vi "GCS26.vi"() -> ()   [LabVIEW 2009]
uses:
  <vilib>/robotics/Controls/Attitude Indicator/Attitude Indicator.xctl
  <vilib>/robotics/Controls/Compass Indicator/Compass Indicator.xctl
  <vilib>/Instr/_visa.llb/VISA Set IO Buffer Mask.ctl
  <vilib>/Instr/_visa.llb/VISA Configure Serial Port (Instr).vi
  user32.dll
panel:
  out "Current Time":string
  out "Compass Indicator":dbl(xcontrol)
  out "Attitude Indicator":cluster{"Roll":dbl, "Pitch":dbl}(xcontrol)
  out "Autopilot switch":bool
  in  "EARTHLib.IKHInterface":refnum<k7>
  out "OriginalChild":i32
  out "TRUE SPEED":dbl(knob) scale=0.0..120.0
  out "COURSE/BEARING":cluster{i16, i16}(knob) scale=0.0..360.0 scale format="%.0f°"
  out "Distance To WP":i32
  out "Current WP":i32
  out "Altitude":cluster{i32, i32}(knob) scale=0.0..200.0
  in  "WebBrowser":refnum<k7>(container)
  out "Air Speed":i32 format="%.0f m/s"
  out "Pitch":i32
  out "Roll":i32
  out "Lat":dbl format="%.6g°"
  out "Lon":dbl format="%.6g°"
  out "Ground Speed":i32 format="%.0f m/s"
  out "C/S Rate\n     Rate":sgl(knob) scale=-5.0..5.0 scale format="%#.2g"
  out "AirSpeed":cluster{i16, i16}(knob)={0, 31} scale=0.0..40.0
  out "Amps":dbl format="%.2f"
  out "Est Time Left":dbl(knob) min=0.0 max=0.0 scale=0.0..60.0 scale format="%#_2f"
  in  "Launch EXE":bool
  out "Watts":dbl format="%.2f"
  out "Slide":u8(slide) scale=0.0..100.0
  out "Throttle S.P":i32 format="%.0f of 100%"
  out "Battery Voltage":dbl format="%#_g V"
  out "LIPO":sgl(slide) scale=9.0..12.6 scale format="%#_g V"
  in  "Logging":bool
  in  "quit?":bool
  in  "Amps FT":i32=34
  in  "MAh's":dbl=2100.0
  in  "Cell Count":dbl=3.0 format="%#_4g"
  out "Boolean 2":bool
  out "Boolean":bool
  in  "Speed":bool
  in  "Baud Rate":string(combo)="38400"
  in  "Choose Port":refnum<visa-resource-name>
  out "error out":errorcluster
  out "Part2":string
  out "Part1":string
  out "ALT":string
  out "originalParent":u32
  in  "EARTHLib.IApplicationGE":refnum<k7>
  in  "WaitForExit":bool
  out "Numeric":i32
  # "C/S Rate"
  # "Air Speed"
  # "Time Left"
  # "Throttle S.P"
  # "LIPO CONDITION"
  # "DIYdrones.com\nEasyuav.com"
  # "ALTITUDE"
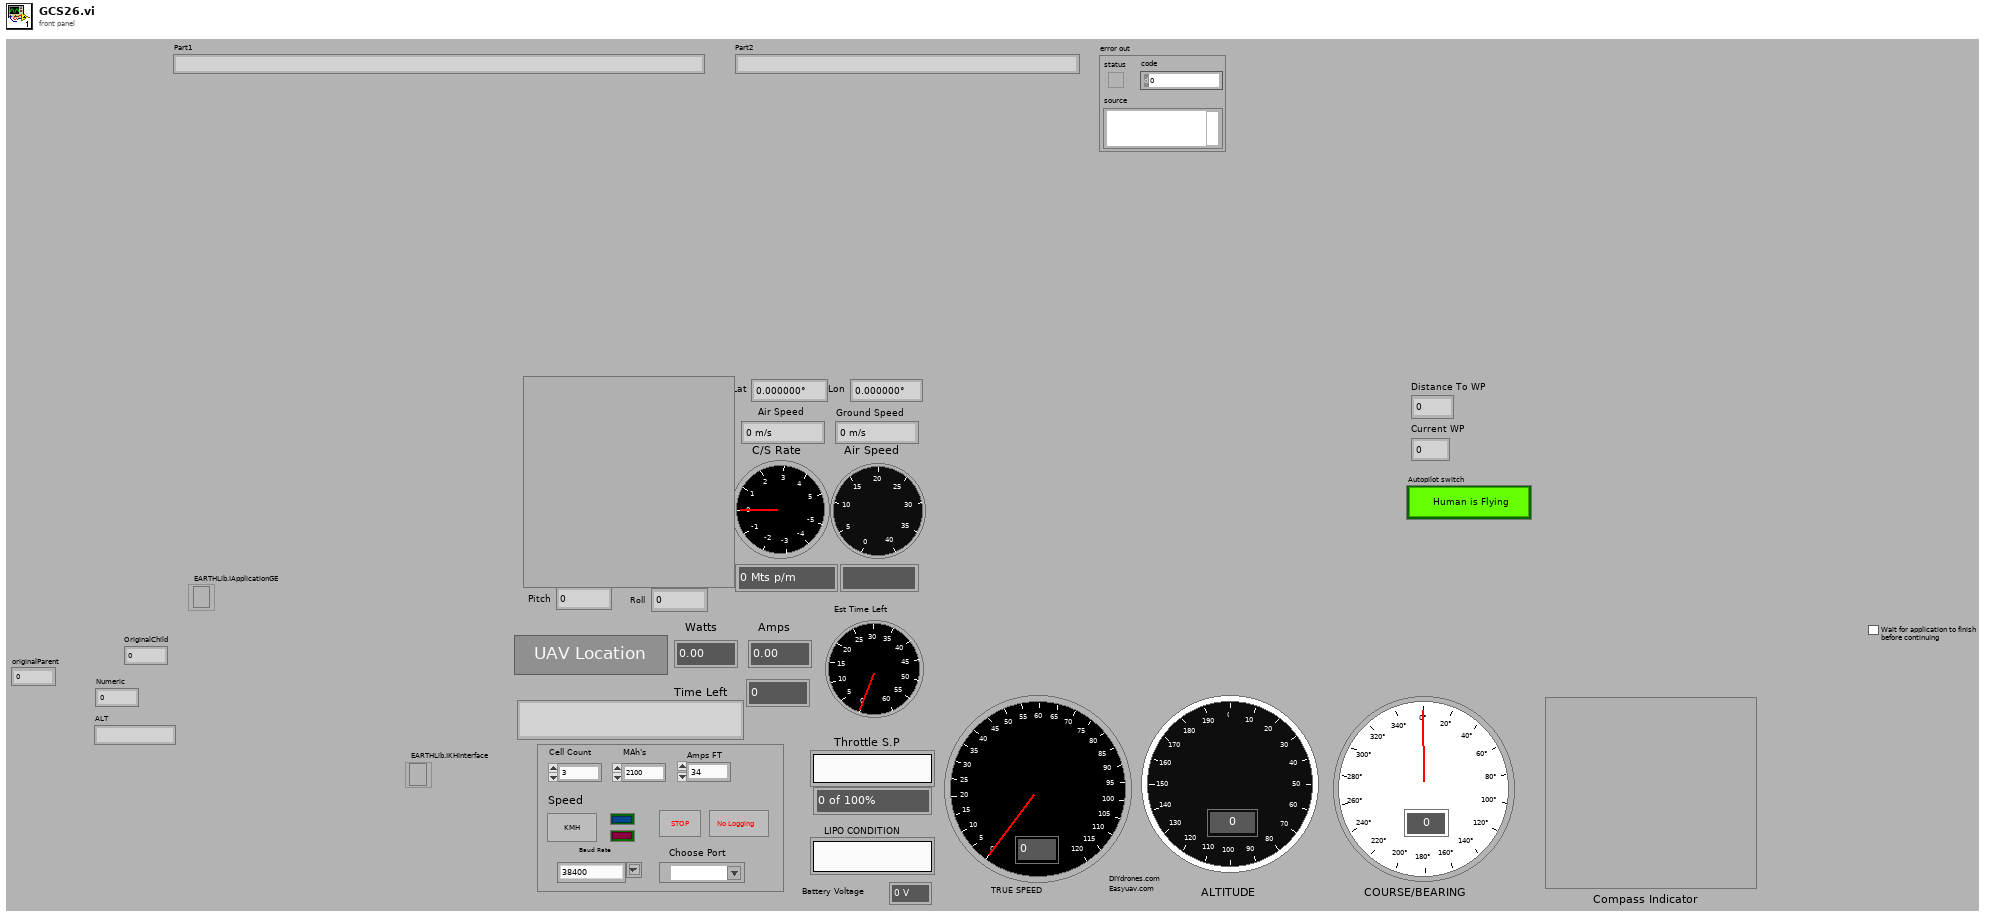
[diagram p1: front panel]
types:
  T1 = enum16{"open", "replace", "create", "open or create", "replace or create", "replace or create with confirmation"}
  T2 = typedef "VISA Set IO Buffer Mask.ctl" = u16
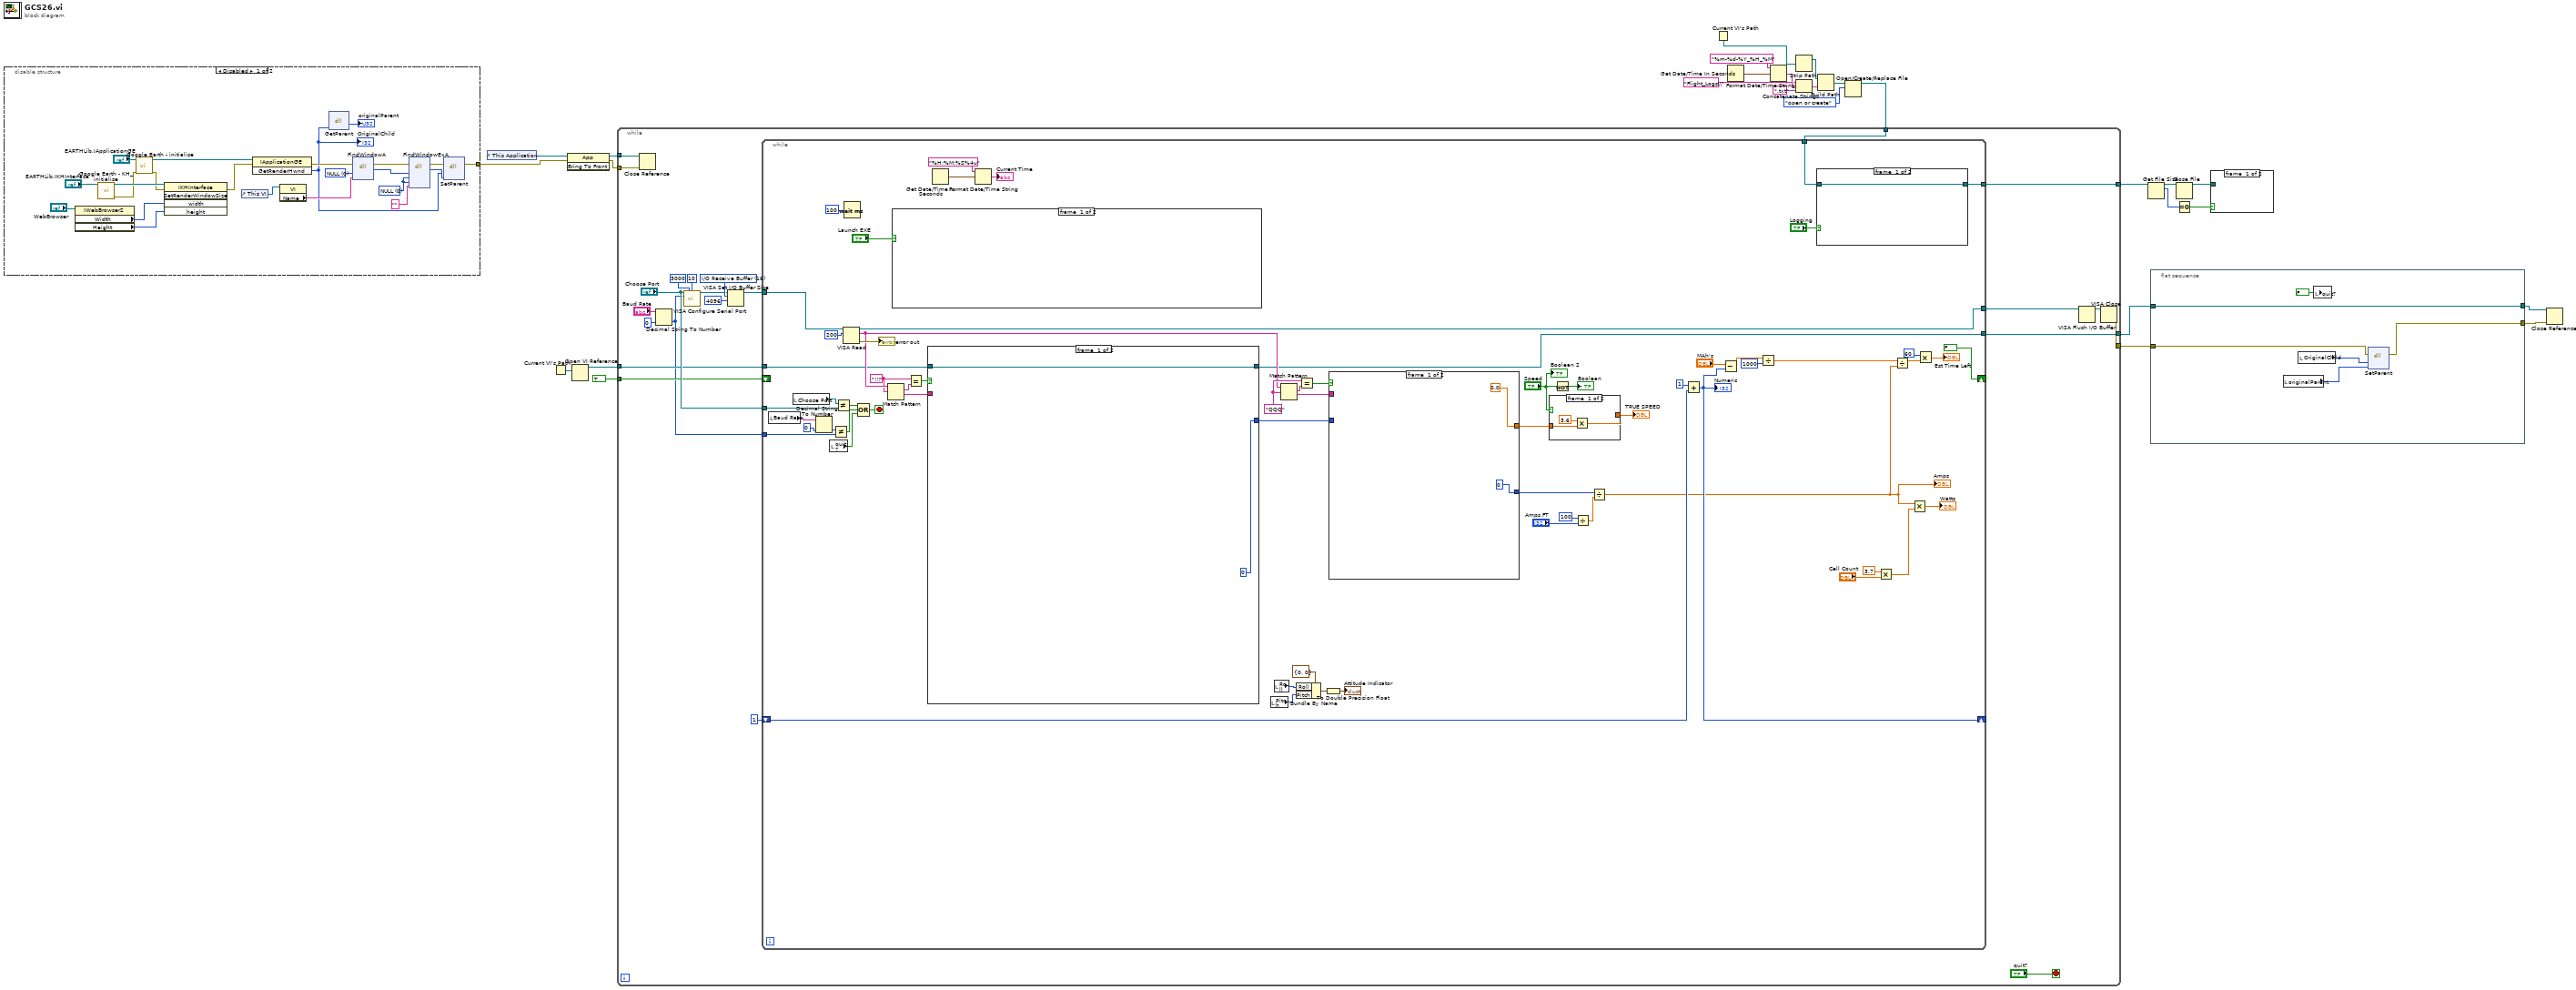
[diagram p0: block diagram]
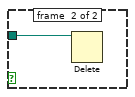
[diagram p2: hidden frame]
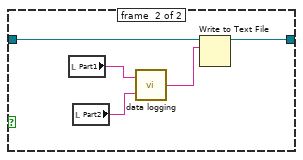
[diagram p4: hidden frame]
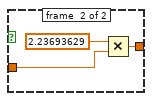
[diagram p5: hidden frame]
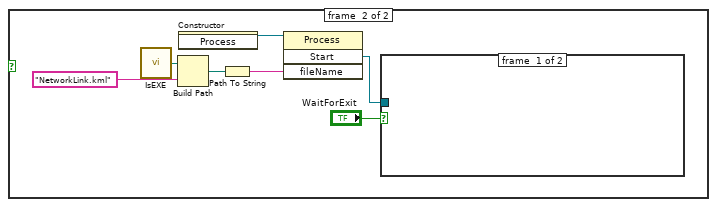
[diagram p6: hidden frame]
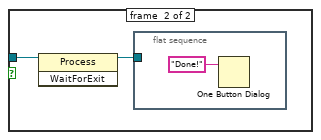
[diagram p7: hidden frame]
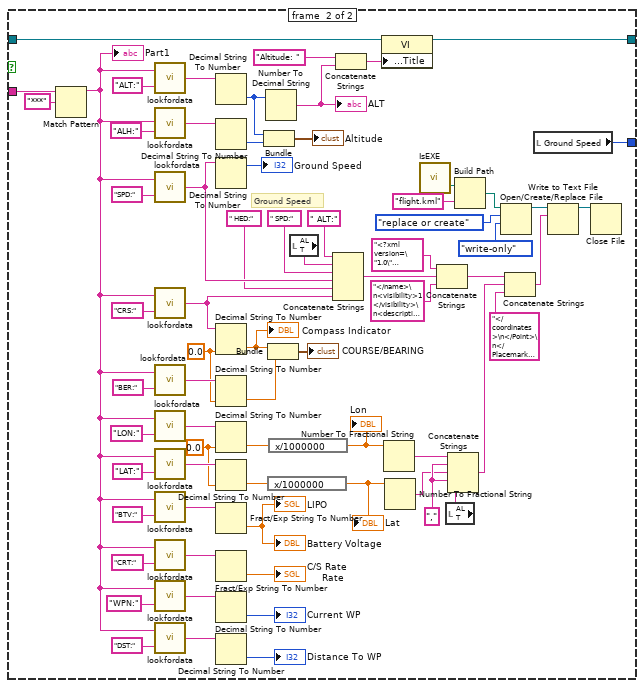
[diagram p8: hidden frame]
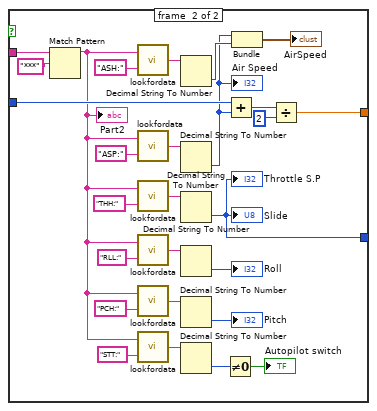
[diagram p9: hidden frame]
diagram:
  n1 = disable-structure shown="Disabled" {
    disable-tunnel: [w29 _] -> w7
    frame #0 {
      w46 = 0 items=["NULL"]
      w48 = 0 items=["NULL"]
      n2 = property class="IWebBrowser2"(reference="WebBrowser") -> ("Width"=w33:i32, "Height"=w32:i32)  [unwired: 1 in, 2 out]
      n3 = call "Google Earth - KH_initialise.vi"("EARTHLib.IKHInterface"="EARTHLib.IKHInterface") -> ("error out"=w28:errorcluster, "Refnum Out"=w34:refnum<k7>)  [unwired: 1 in, 8 out]
      n4 = call "Google Earth - initialise.vi"("error in (no error)"=w28, "EARTHLib.IApplicationGE"="EARTHLib.IApplicationGE") -> ("error out"=w31:errorcluster, "Refnum Out"=w49:refnum<k7>)  [unwired: 8 out]
      n5 = invoke class="IKHInterface" method="SetRenderWindowSize"(reference=w34, error in=w31, "width"=w33, "height"=w32) -> (error out=w30:errorcluster)  [unwired: 1 in, 4 out]
      n6 = control-ref of="This VI"() -> (w40:refnum<vi>)
      n7 = invoke class="IApplicationGE" method="GetRenderHwnd"(reference=w49, error in=w30) -> (error out=w37:errorcluster, "GetRenderHwnd"=w36:i32)  [unwired: 1 in, 1 out]
      "OriginalChild" <- w36
      n8 = property class="VI"(reference=w40) -> ("Name"=w39:string)  [unwired: 1 in, 2 out]
      n9 = dll-call lib="user32.dll" fn="GetParent" label="Get Parent"("hWndChild"=w36) -> ("hWnd"=→"originalParent":u32)  [unwired: 4 in, 2 out]
      n10 = dll-call lib="user32.dll" fn="FindWindowA" label="FindWindow"(error in=w37, "lpszClassName"=w48, "lpszWindowName"=w39) -> (error out=w43:errorcluster, "hWnd"=w47:u32)  [unwired: 4 in, 1 out]
      n11 = dll-call lib="user32.dll" fn="FindWindowExA" label="Find Child"(error in=w43, "Parent HWND"=w47, "Child_After HWND"=w46, "lpszClassName"=w46, "lpszWindowName"="") -> (error out=w41:errorcluster, "hWnd"=w45:u32)  [unwired: 5 in, 2 out]
      n12 = dll-call lib="user32.dll" fn="SetParent" label="Set Parent"(error in=w41, "hWndChild"=w36, "hWndNewParent"=w45) -> (error out=w29:errorcluster)  [unwired: 4 in, 2 out]
    }
    frame #1 {
    }
  }
  n13 = control-ref of="This Application"() -> (w20:refnum<vi>)
  n14 = Current VI's Path() -> (path=w26:path)
  n15 = invoke class="App" method="Bring To Front"(reference=w20, error in=w7) -> (reference out=w19:refnum<vi>, error out=w18:errorcluster)  [unwired: 1 in, 1 out]
  n16 = Open VI Reference(vi path=w26) -> (vi reference=w25:refnum<vi>)  [unwired: 1 in, 5 out]
  n17 = Current VI's Path() -> (path=w9:path)
  n18 = Get Date/Time In Seconds() -> (seconds since 1Jan1904=w12:timestamp)
  n19 = Format Date/Time String(time format string (%c)="%m-%d-%Y_%H_%M", seconds (now)=w12) -> (date/time string=w11:string)  [unwired: 1 out]
  n20 = Strip Path(path=w9) -> (stripped path=w8:path)  [unwired: 1 out]
  n21 = Concatenate Strings("Flight_Logs\\" ("string"), w11, ".txt" ("string")) -> (w17:string)
  n22 = Build Path(base path=w8, name or relative path=w17) -> (appended path=w15:path)
  n23 = Open/Create/Replace File(file path (use dialog)=w15, operation (0:open)=T1."open or create") -> (refnum out=w14:refnum<file>)  [unwired: 1 in, 5 out]
  n24 = while {
    tunnel: TRUE -> [w63]
    tunnel: [w62] -> w24
    tunnel: w25 -> [w61]
    tunnel: [w57] -> w21
    tunnel: w19 -> [w56]
    tunnel: w18 -> [w55]
    tunnel: [w54] -> w5
    tunnel: w14 -> [w53]
    stop <- "quit?" stop-if-true
    w72 = T2 16 items=["I/O Receive Buffer"=16, "I/O Transmit Buffer"=32, "I/O Receive and Transmit Buffer"=48] ("Mask")
    n25 = Close Reference(reference=w56, error in (no error)=w55) -> ()  [unwired: 1 out]
    n26 = Decimal String To Number(string="Baud Rate", default (0L)=u32 0 ("default (0 I32)")) -> (number=w52:u32)  [unwired: 2 out]
    n27 = call-poly "VISA Configure Serial Port"("VISA resource name"="Choose Port", "timeout (10sec)"=u32 3000, "termination char\n(0xA = '\\n' = LF)"=u8 10 ("termination char\n(0xA = '\\n' = LF)"), "baud rate (9600)"=w52) -> ("VISA resource name out"=w65:refnum<visa-resource-name>)  [unwired: 5 in, 6 out]
    n28 = VISA Set I/O Buffer Size(VISA resource name=w65, mask (16)=w72, size (4096)=u32 4096) -> (VISA resource name out=w70:refnum<visa-resource-name>)  [unwired: 1 in, 1 out]
    n29 = while {
      tunnel: w70 -> [w134]
      tunnel: [w133] -> w69
      tunnel: "Choose Port" -> [w123]
      shift-right: [FALSE] -> _
      shift-left: w63 -> [_]
      tunnel: [w121] -> w62
      tunnel: w61 -> [w120]
      tunnel: w52 -> [w119]
      shift-right: [w102] -> _
      shift-left: 1 ("Slide 2") -> [w113]
      tunnel: [w88] -> w54
      tunnel: w53 -> [w87]
      stop <- w116 stop-if-true
      w128 = "QQQ" ("regular expression")
      w76 = "!!!" ("regular expression")
      n30 = local read "Baud Rate"() -> (w115:string)
      n31 = local read "Choose Port"() -> (w124:refnum<visa-resource-name>)
      n32 = Decimal String To Number(string=w115, default (0L)=u32 0 ("default (0 I32)")) -> (number=w74:u32)  [unwired: 2 out]
      n33 = local read "quit?"() -> (w90:bool)
      n34 = Not Equal?(x=w74, y=w119) -> (x != y?=w117:bool)
      n35 = Not Equal?(x=w124, y=w123) -> (x != y?=w118:bool)
      n36 = VISA Read(VISA resource name=w134, byte count=u32 200) -> (VISA resource name out=w133:refnum<visa-resource-name>, read buffer=w126:string, error out=→"error out":errorcluster)  [unwired: 1 in, 1 out]
      n37 = Wait (ms)(milliseconds to wait=u32 100) -> ()  [unwired: 1 out]
      n38 = Compound Arithmetic op=OR(w118, w117, w90) -> (w116:bool)
      n39 = Match Pattern(string=w126, regular expression=w76) -> (match substring=w75:string, after substring=w135:string)  [unwired: 3 out]
      n40 = case shown="True" "Launch EXE" {
        frame #0 {
        }
        frame #1 {
          n41 = call "IsEXE.vi"() -> ("path to vi or exe install\\data\\ dir"=w148:path)  [unwired: 10 out]
          n42 = Build Path(base path=w148, name or relative path="NetworkLink.kml") -> (appended path=w149:path)
          n43 = constructor class="Process"() -> (reference out=w154:refnum<k24>)  [unwired: 3 in, 2 out]
          n44 = Path To String(path=w149) -> (string=w153:string)
          n45 = invoke class="Process" method="Start"(reference=w154, "fileName"=w153) -> ("Start"=w152:refnum<k24>)  [unwired: 2 in, 3 out]
          n46 = case shown="True" "WaitForExit" {
            tunnel: w152 -> [_ w156]
            frame #0 {
            }
            frame #1 {
              n47 = invoke class="Process" method="WaitForExit"(reference=w156) -> (reference out=w155:refnum<k24>)  [unwired: 2 in, 2 out]
              n48 = flat-sequence {
                tunnel: w155 -> [_]
                frame #0 {
                  n49 = One Button Dialog(message="Done!") -> ()  [unwired: 2 out]
                }
              }
            }
          }
        }
      }
      n50 = Equal?(x=w76, y=w75) -> (x = y?=w106:bool)
      n51 = case shown="True" w106 {
        tunnel: w135 -> [_ w187]
        tunnel: [w158 w184] -> w121
        tunnel: w120 -> [w158 w161]
        tunnel: [0 ("Numeric") w173] -> w112
        frame #0 {
        }
        frame #1 {
          w162 = 0.0 ("default (0 I32)")
          w163 = 0.0 ("default (0 I32)")
          w176 = ","
          # "Ground Speed"
          n52 = Match Pattern(string=w187, regular expression="***") -> (before substring=w168:string)  [unwired: 4 out]
          "Part1" <- w168
          n53 = call "lookfordata.vi"("Header"="ALT:" ("regular expression"), "string"=w168) -> ("output string"=w160:string)
          n54 = call "lookfordata.vi"("Header"="ALH:" ("regular expression"), "string"=w168) -> ("output string"=w225:string)
          n55 = call "lookfordata.vi"("Header"="SPD:", "string"=w168) -> ("output string"=w194:string)
          n56 = call "lookfordata.vi"("Header"="CRS:", "string"=w168) -> ("output string"=w191:string)
          n57 = call "lookfordata.vi"("Header"="BER:", "string"=w168) -> ("output string"=w223:string)
          n58 = call "lookfordata.vi"("Header"="LON:", "string"=w168) -> ("output string"=w213:string)
          n59 = call "lookfordata.vi"("Header"="LAT:", "string"=w168) -> ("output string"=w211:string)
          n60 = call "lookfordata.vi"("Header"="BTV:", "string"=w168) -> ("output string"=w181:string)
          n61 = call "lookfordata.vi"("Header"="CRT:", "string"=w168) -> ("output string"=w189:string)
          n62 = call "lookfordata.vi"("Header"="WPN:", "string"=w168) -> ("output string"=w219:string)
          n63 = call "lookfordata.vi"("Header"="DST:", "string"=w168) -> ("output string"=w209:string)
          n64 = Decimal String To Number(string=w160) -> (number=w178:i32)  [unwired: 3 out]
          n65 = Decimal String To Number(string=w225) -> (number=w226:i32)  [unwired: 3 out]
          n66 = Decimal String To Number(string=w194) -> (offset past number=→"Ground Speed":i32)  [unwired: 3 out]
          n67 = Decimal String To Number(string=w191, default (0L)=w162) -> (number=w166:dbl)  [unwired: 2 out]
          "Compass Indicator" <- w166
          n68 = Decimal String To Number(string=w223, default (0L)=w162) -> (number=w224:dbl)  [unwired: 2 out]
          n69 = Decimal String To Number(string=w213, default (0L)=w163) -> (number=w165:dbl)  [unwired: 2 out]
          n70 = Decimal String To Number(string=w211, default (0L)=w163) -> (number=w164:dbl)  [unwired: 2 out]
          n71 = Fract/Exp String To Number(string=w181) -> (number=→"LIPO" →"Battery Voltage":dbl)  [unwired: 4 out]
          n72 = Fract/Exp String To Number(string=w189) -> (number=→"C/S Rate\n     Rate":dbl)  [unwired: 4 out]
          n73 = Decimal String To Number(string=w219) -> (number=→"Current WP":i32)  [unwired: 3 out]
          n74 = Decimal String To Number(string=w209) -> (number=→"Distance To WP":i32)  [unwired: 3 out]
          n75 = Bundle(w178, w226) -> (→"Altitude":cluster{i32, i32})  [unwired: 1 out]
          n76 = Number To Decimal String(number=w178) -> (decimal integer string=w172:string)  [unwired: 1 out]
          "ALT" <- w172
          n77 = Bundle(w166, w224) -> (→"COURSE/BEARING":cluster{dbl, dbl})  [unwired: 1 out]
          n78 = expression code="x/1000000"(w164) -> (w199:dbl)
          "Lat" <- w199
          n79 = expression code="x/1000000"(w165) -> (w200:dbl)
          "Lon" <- w200
          n80 = local read "ALT"() -> (w171:string)
          n81 = Concatenate Strings(" ALT:", w171, " SPD:", w194, " HED:", w191) -> (w167:string)
          n82 = Concatenate Strings("Altitude: " ("string"), w172) -> (w185:string)
          n83 = property class="VI"(reference=w161, "Front Panel.Title"=w185) -> (reference out=w184:refnum<vi>)  [unwired: 1 in, 1 out]
          n84 = Number To Fractional String(number=w200) -> (F-format string=w175:string)  [unwired: 3 out]
          n85 = Number To Fractional String(number=w199) -> (F-format string=w174:string)  [unwired: 3 out]
          n86 = call "IsEXE.vi"() -> ("path to vi or exe install\\data\\ dir"=w186:path)  [unwired: 10 out]
          n87 = Concatenate Strings("<?xml version=\"1.0\" encoding=\"UTF-8\"?>\n<kml xmlns=\"http://www.opengis.net/kml/2.2\">\n<Placemark>\n<name>", w167, "</name>\n<visibility>1</visibility>\n<description>Current Position</description>\n<Style>\n<IconStyle>\n<Icon>\n<href>http://maps.google.com/mapfiles/kml/shapes/airports.png</href>\n</Icon>\n</IconStyle>\n<LineStyle>\n<width>2</width>\n</LineStyle>\n</Style>\n<Point>\n<extrude>1</extrude>\n<altitudeMode>relativeToGround</altitudeMode>\n<coordinates>") -> (w196:string)
          n88 = local read "ALT"() -> (w170:string)
          n89 = Concatenate Strings(w175, w176, w174, w176, w170) -> (w169:string)
          n90 = Build Path(base path=w186, name or relative path="flight.kml") -> (appended path=w207:path)
          n91 = Open/Create/Replace File(file path (use dialog)=w207, operation (0:open)=T1."replace or create", access (0:read/write)=enum16{"read/write", "read-only", "write-only"}."write-only") -> (refnum out=w203:refnum<file>)  [unwired: 1 in, 4 out]
          n92 = Concatenate Strings(w196, w169, "</coordinates>\n</Point>\n</Placemark>\n</kml>") -> (w202:string)
          n93 = local read "Ground Speed"() -> (w173:i32)
          n94 = Write to Text File(file (use dialog)=w203, text=w202) -> (refnum out=w201:refnum<file>)  [unwired: 1 in, 3 out]
          n95 = Close File(refnum=w201) -> ()  [unwired: 1 in, 2 out]
        }
      }
      n96 = Get Date/Time In Seconds() -> (seconds since 1Jan1904=w78:timestamp)
      n97 = Format Date/Time String(time format string (%c)="%H:%M:%S%4u", seconds (now)=w78) -> (date/time string=→"Current Time":string)  [unwired: 1 out]
      n98 = local read "Pitch"() -> (w80:i32)
      n99 = local read "Roll"() -> (w81:i32)
      n100 = Match Pattern(string=w126, regular expression=w128) -> (match substring=w127:string, after substring=w129:string)  [unwired: 3 out]
      n101 = Bundle By Name(cluster=cluster{"Roll":i32, "Pitch":i32} {"Roll"=0, "Pitch"=0} ("Attitude Indicator"), "Roll"=w81, "Pitch"=w80) -> (w83:cluster{"Roll":i32, "Pitch":i32})
      n102 = Equal?(x=w128, y=w127) -> (x = y?=w110:bool)
      n103 = To Double Precision Float(number=w83) -> (double precision float=→"Attitude Indicator":cluster{"Roll":dbl, "Pitch":dbl})
      n104 = case shown="True" w110 {
        tunnel: w129 -> [_ w250]
        tunnel: w112 -> [_ w246]
        tunnel: [0.0 w244] -> w109
        tunnel: [0 w243] -> w91
        frame #0 {
        }
        frame #1 {
          n105 = Match Pattern(string=w250, regular expression="***") -> (before substring=w235:string)  [unwired: 4 out]
          "Part2" <- w235
          n106 = call "lookfordata.vi"("Header"="ASH:" ("regular expression"), "string"=w235) -> ("output string"=w256:string)
          n107 = call "lookfordata.vi"("Header"="ASP:" ("regular expression"), "string"=w235) -> ("output string"=w242:string)
          n108 = call "lookfordata.vi"("Header"="THH:" ("regular expression"), "string"=w235) -> ("output string"=w254:string)
          n109 = call "lookfordata.vi"("Header"="RLL:", "string"=w235) -> ("output string"=w241:string)
          n110 = call "lookfordata.vi"("Header"="PCH:", "string"=w235) -> ("output string"=w240:string)
          n111 = call "lookfordata.vi"("Header"="STT:", "string"=w235) -> ("output string"=w234:string)
          n112 = Decimal String To Number(string=w256) -> (number=w257:i32)  [unwired: 3 out]
          n113 = Decimal String To Number(string=w242) -> (number=w245:i32)  [unwired: 3 out]
          "Air Speed" <- w245
          n114 = Decimal String To Number(string=w254) -> (number=w243:i32)  [unwired: 3 out]
          "Throttle S.P" <- w243
          "Slide" <- w243
          n115 = Decimal String To Number(string=w241) -> (number=→"Roll":i32)  [unwired: 3 out]
          n116 = Decimal String To Number(string=w240) -> (number=→"Pitch":i32)  [unwired: 3 out]
          n117 = Decimal String To Number(string=w234) -> (number=w233:i32)  [unwired: 3 out]
          n118 = Not Equal To 0?(x=w233) -> (x != 0?=→"Autopilot switch":bool)
          n119 = Add(x=w246, y=w245) -> (x+y=w247:i32)
          n120 = Bundle(w245, w257) -> (→"AirSpeed":cluster{i32, i32})  [unwired: 1 out]
          n121 = Divide(x=w247, y=2) -> (x/y=w244:dbl)
        }
      }
      n122 = case shown="True" "Speed" {
        tunnel: [w143 w146] -> w111
        tunnel: w109 -> [w142 w145]
        frame #0 {
          n123 = Multiply(x=3.6, y=w142) -> (x*y=w143:dbl)
        }
        frame #1 {
          n124 = Multiply(x=2.23693629, y=w145) -> (x*y=w146:dbl)
        }
      }
      "TRUE SPEED" <- w111
      n125 = Not(x="Speed") -> (.not. x?=→"Boolean":bool)
      n126 = Divide(x=100 ("Slide 2"), y="Amps FT") -> (x/y=w92:dbl)
      n127 = Divide(x=w91, y=w92) -> (x/y=w86:dbl)
      "Amps" <- w86
      n128 = Add(x=1, y=w113) -> (x+y=w102:i32)
      "Numeric" <- w102
      n129 = Subtract(x="MAh's", y=w102) -> (x-y=w97:dbl)
      n130 = Divide(x=w97, y=1000 ("Slide 2")) -> (x/y=w95:dbl)
      n131 = case shown="True" "Logging" {
        tunnel: [w136 w141] -> w88
        tunnel: w87 -> [w136 w139]
        frame #0 {
        }
        frame #1 {
          n132 = local read "Part1"() -> (w138:string)
          n133 = local read "Part2"() -> (w137:string)
          n134 = call "data logging.vi"("Part1 2"=w137, "Part1"=w138) -> ("Output String"=w140:string)
          n135 = Write to Text File(file (use dialog)=w139, text=w140) -> (refnum out=w141:refnum<file>)  [unwired: 1 in, 3 out]
        }
      }
      n136 = Multiply(x=3.7, y="Cell Count") -> (x*y=w85:dbl)
      n137 = Divide(x=w95, y=w86) -> (x/y=w99:dbl)
      n138 = Multiply(x=w86, y=w85) -> (x*y=→"Watts":dbl)
      n139 = Multiply(x=60 ("Slide 2"), y=w99) -> (x*y=→"Est Time Left":dbl)
      "Boolean 2" <- "Speed"
    }
    n140 = VISA Flush I/O Buffer(VISA resource name=w69) -> (VISA resource name out=w68:refnum<visa-resource-name>)  [unwired: 1 in, 2 out]
    n141 = VISA Close(VISA resource name=w68) -> (error out=w57:errorcluster)  [unwired: 1 in]
  }
  n142 = Get File Size(file=w5) -> (refnum out=w2:refnum<file>, size (in bytes)=w3:i64)  [unwired: 1 in, 1 out]
  n143 = flat-sequence {
    tunnel: w24 -> [w264]
    tunnel: [w264] -> w23
    tunnel: [w261] -> w22
    tunnel: w21 -> [w260]
    frame #0 {
      n144 = local read "originalParent"() -> (w262:u32)
      n145 = local read "OriginalChild"() -> (w259:i32)
      n146 = local write "quit?"(FALSE ("quit?")) -> ()
      n147 = dll-call lib="user32.dll" fn="SetParent" label="Set Parent"(error in=w260, "hWndChild"=w259, "hWndNewParent"=w262) -> (error out=w261:errorcluster)  [unwired: 4 in, 2 out]
    }
  }
  n148 = Close File(refnum=w2) -> (path=w1:path)  [unwired: 1 in, 1 out]
  n149 = Equal To 0?(x=w3) -> (x = 0?=w4:bool)
  n150 = case shown="True" w4 {
    tunnel: w1 -> [_ w265]
    frame #0 {
    }
    frame #1 {
      n151 = Delete(path (use dialog)=w265) -> ()  [unwired: 4 in, 3 out]
    }
  }
  n152 = Close Reference(reference=w23, error in (no error)=w22) -> ()  [unwired: 1 out]
